vi "Core Action.vi"(8 "error in (no error)":errorcluster, 10 "SECS-II Class":refnum<class "SECS-II Class.lvclass">, 11 "27-Host Requests to Enter On-Line in":refnum<class "27-Host Requests to Enter On-Line.lvclass">) -> (0 "error out":errorcluster, 2 "SECS-II Class Out":refnum<class "SECS-II Class.lvclass">, 3 "27-Host Requests to Enter On-Line out":refnum<class "27-Host Requests to Enter On-Line.lvclass">)   [LabVIEW 2020, in "SECS Scenarios.lvlib" / "27-Host Requests to Enter On-Line.lvclass"]
uses:
  27-Host Requests to Enter On-Line.lvclass
  D:/Dropbox/SECS/SECS_GEM v1.1.0/Com/SECS Scenarios/Scenarios Class/Scenarios Class.lvclass
  SECS Communication/SECS-II Class/SECS-II Class.lvclass
  SECS Communication/S1 Message Class/S1 Message Class.lvclass
  D:/Dropbox/SECS/SECS_GEM v1.1.0/Com/SECS Communication/SECS-II Class/SECS-II Class.lvclass
  Scenarios Class/Reply State.ctl
  Scenarios Class/Scenarios Class.lvclass/Scenarios Class.ctl
  Scenarios Class/Write Reply State.vi
  Scenarios Class/Read HSMS Class.vi
  SECS Communication/HSMS Class/HSMS Class.lvclass
  Scenarios Class/Scenarios Class.lvclass
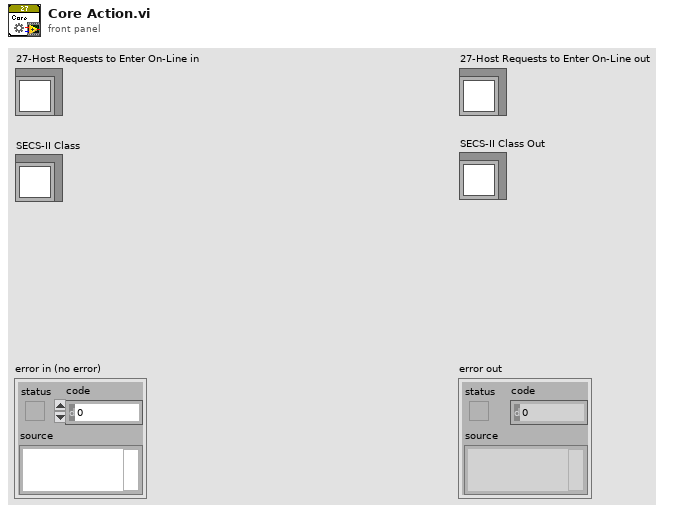
[diagram p1: front panel]
types:
  T1 = typedef "SECS Scenarios.lvlib/Scenarios Class.lvclass/Reply State.ctl" = enum16{"OK", "Illegal Data", "Unknown Stream", "Unknown Function", "Off-Line", "T3 Timeout", "Inner-Timeout"}
  T2 = typedef "SECS Communication.lvlib/S1 Message Class.lvclass/S1F18.ctl" = enum16{"ok", "refused", "already online"}
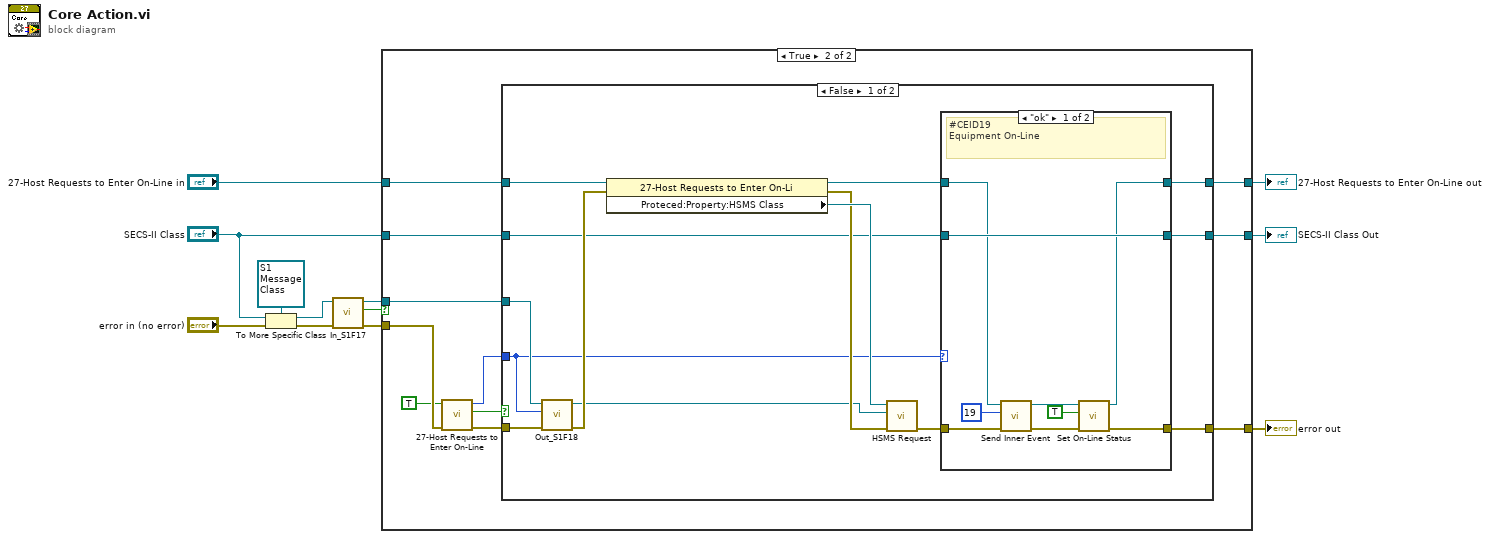
[diagram p0: block diagram]
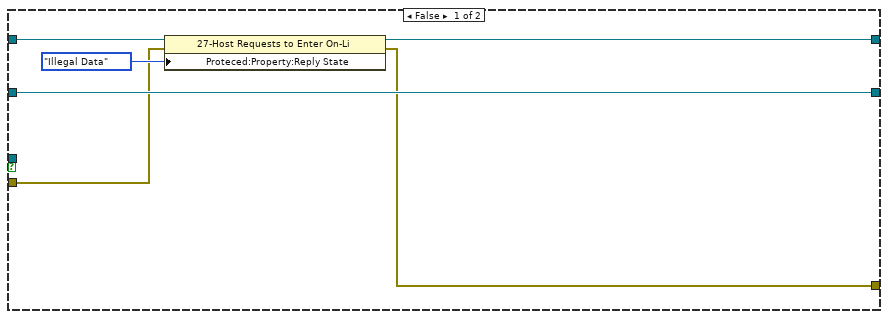
[diagram p2: hidden frame]
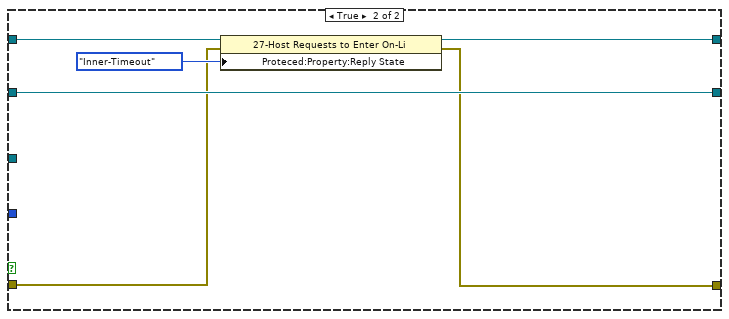
[diagram p4: hidden frame]
diagram:
  n1 = To More Specific Class(target class=refnum<class "S1 Message Class.lvclass"> refnum ("SECS Communication.lvlib:S1 Message Class.lvclass"), reference="SECS-II Class", error in="error in (no error)") -> (specific class reference=w11:refnum<class "S1 Message Class.lvclass">, error out=w12:errorcluster)
  n2 = call "In_S1F17.vi"("error in (no error)"=w12, "S1 Message Class in"=w11) -> ("error out"=w3:errorcluster, "OK?"=w2:bool, "S1 Message Class out"=w10:refnum<class "S1 Message Class.lvclass">)  [unwired: 7 in]
  n3 = case shown="True" w2 {
    tunnel: w10 -> [_ w29]
    tunnel: "27-Host Requests to Enter On-Line in" -> [w18 w28]
    tunnel: [w13 w27] -> w6
    tunnel: [w17 w26] -> w1
    tunnel: "SECS-II Class" -> [w16 w25]
    tunnel: [w16 w24] -> w4
    tunnel: w3 -> [w14 w20]
    frame False {
      n4 = property class="27-Host Requests to Enter On-Li"(reference=w18, error in=w14, "Proteced:Property:Reply State"=Reply_State."Illegal Data" ("Reply State")) -> (reference out=w17:refnum<class "27-Host Requests to Enter On-Line.lvclass">, error out=w13:errorcluster)
    }
    frame True {
      n5 = call "27-Host Requests to Enter On-Line.vi"("error in (no error)"=w20, "On-Line"=TRUE) -> ("error out"=w23:errorcluster, "Timeout?"=w22:bool, "S1F18"=w21:T2)  [unwired: 7 in]
      n6 = case shown="False" w22 {
        tunnel: w28 -> [w43 w59]
        tunnel: w29 -> [w40 _]
        tunnel: [w34 w56] -> w27
        tunnel: [w32 w57] -> w26
        tunnel: w23 -> [w37 w58]
        tunnel: w21 -> [w35 _]
        tunnel: w25 -> [w31 w61]
        tunnel: [w30 w61] -> w24
        frame False {
          n7 = call "Out_S1F18.vi"("error in (no error)"=w37, "S1F18"=w35, "S1 Message Class in"=w40) -> ("error out"=w39:errorcluster, "S1 Message Class out"=w38:refnum<class "S1 Message Class.lvclass">)  [unwired: 7 in]
          n8 = property class="27-Host Requests to Enter On-Li"(reference=w43, error in=w39) -> (reference out=w33:refnum<class "27-Host Requests to Enter On-Line.lvclass">, error out=w41:errorcluster, "Proteced:Property:HSMS Class"=w42:refnum<class "HSMS Class.lvclass">)
          n9 = call "HSMS Request.vi"("error in (no error)"=w41, "SECS-II Class In"=w38, "HSMS Class in"=w42) -> ("error out"=w36:errorcluster)  [unwired: 7 in, 1 out]
          n10 = case shown="\"ok\"" w35 {
            tunnel: w36 -> [w48 w55]
            tunnel: [w49 w55] -> w34
            tunnel: w33 -> [w47 w54]
            tunnel: [w50 w54] -> w32
            tunnel: w31 -> [w52 w53]
            tunnel: [w52 w53] -> w30
            frame "ok" {
              # "#CEID19\nEquipment On-Line"
              n11 = call "Send Inner Event.vi"("error in (no error)"=w48, "CEID"=u32 19, "Scenarios Class in"=w47) -> ("error out"=w45:errorcluster, "Scenarios Class out"=w46:refnum<class "27-Host Requests to Enter On-Line.lvclass">)  [unwired: 7 in]
              n12 = call "Set On-Line Status.vi"("error in (no error)"=w45, "On-Line"=TRUE ("On-Line Status"), "Scenarios Class in"=w46) -> ("error out"=w49:errorcluster, "Scenarios Class out"=w50:refnum<class "27-Host Requests to Enter On-Line.lvclass">)  [unwired: 7 in]
            }
            frame Default {
            }
          }
        }
        frame True {
          n13 = property class="27-Host Requests to Enter On-Li"(reference=w59, error in=w58, "Proteced:Property:Reply State"=Reply_State."Inner-Timeout" ("Reply State")) -> (reference out=w57:refnum<class "27-Host Requests to Enter On-Line.lvclass">, error out=w56:errorcluster)
        }
      }
    }
  }
  "error out" <- w6
  "27-Host Requests to Enter On-Line out" <- w1
  "SECS-II Class Out" <- w4
